vi "Scale Byte TB.vi"() -> ()   [LabVIEW 2013]
panel:
  out "Scaled Color":i32[][](array[numeric])
  in  "Brightness":u8
  in  "Factor":dbl
  in  "stop":bool
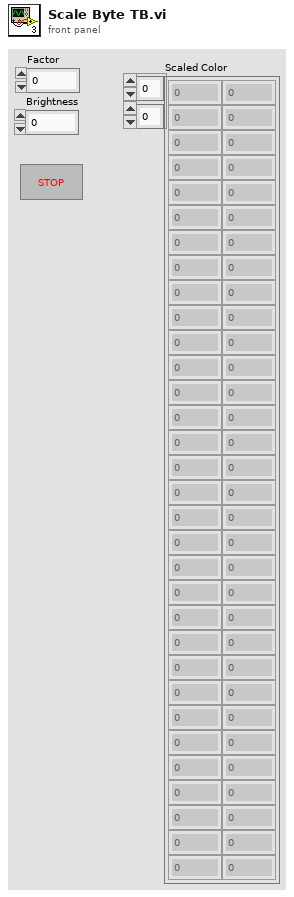
[diagram p1: front panel]
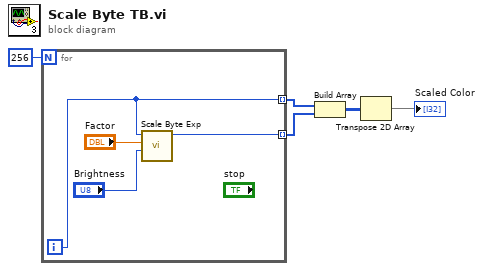
[diagram p0: block diagram]
diagram:
  n1 = for {
    N: 256 -> [_]
    tunnel: [w7] -> w3 mode=indexing
    tunnel: [w6] -> w4 mode=indexing
    i -> [w6]
    n2 = call "Scale Byte Exp.vi"("Brightness"="Brightness", "Factor"="Factor", "Byte"=w6) -> ("Byte Scaled"=w7:u8)  [unwired: 8 in]
  }
  n3 = Build Array(w4, w3) -> (w2:i32[][])
  n4 = Transpose 2D Array(2D array=w2) -> (transposed array=→"Scaled Color":i32[][])
